vi "MAIN_save_merFISH_setpoint.vi"(3 "error in":errorcluster, 4 "Start acquisition":bool) -> (0 "error out":errorcluster, 1 "Next task":T2, 2 "QPD":T1)   [LabVIEW 2015]
uses:
  CONTROLS/Q_main_element.ctl
  GLOBAL/Global_FPGA.vi
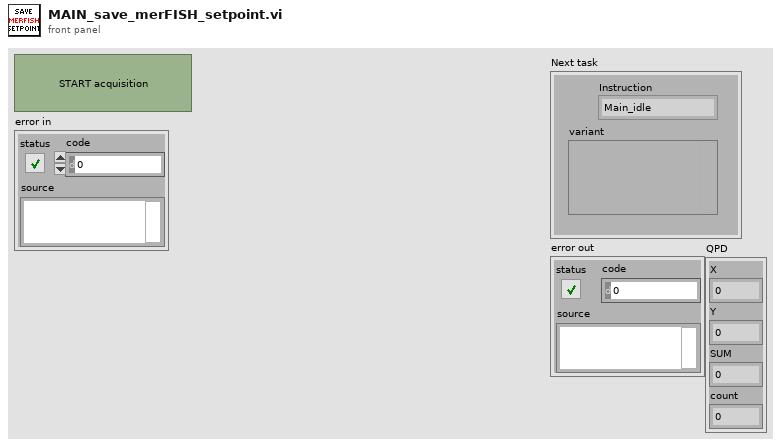
[diagram p1: front panel]
types:
  T1 = cluster{"X":sgl, "Y":sgl, "SUM":sgl, "count":u32}
  T2 = typedef "Q_main_element.ctl" = cluster{"variant":variant, "Instruction":enum16{"Main_idle", "Main_initialize", "Main_initialize_TDMS", "Main_initialize_Queue", "Main_error", "Main_DAQ_initialization_results", "Main_ASI_initialization_results", "Main_Piezo_initialization_results", "Main_Valve_initialization_results", "Main_Pump_initialization_results", "Main_CAMERA_initialization_results", "Main_FPGA_initialization_results", "Main_DAQ_error", "Main_ASI_error", "Main_Piezo_error", "Main_CAMERA_error", "Main_Valve_error", "Main_Pump_error", "Main_FPGA_error", "Main_start_acquiring", "Main_not_acquiring", "Main_acquiring", "Main_stop_acquiring", "Main_change_exposure", "Main_change_z_scan_parameters", "Main_define_ROI", "Main_define_mosaic", "Main_read_kinetic_time", "Main_cooler", "Main_read_temperature", "Main_save_XY", "Main_load_XY", "Main_discard_XY", "Main_move_to_XY", "Main_measure_QPD", "Main_autofocus_calibration", "Main_autofocus_initialization", "Main_autofocus_stop", "Main_save_PID", "Main_change_H_valve_position", "Main_two_way_valve", "Main_save_movie", "Main_init_single_scan", "Main_single_scan", "Main_stop_single_scan", "Main_merFISH_illumination_parameters", "Main_merFISH_buffer_probe_list", "Main_merFISH_injections_procedure", "Main_merFISH_save_setpoint", "Main_merFISH_DAPI_parameters", "Main_merFISH_Brightfield_parameters", "Main_merFISH_save_embryo_ROI", "Main_merFISH_init", "Main_merFISH_resume", "Main_merFISH_start_autofocus", "Main_merFISH_open_close_valve_merFISH", "Main_merFISH_open_close_valve_photobleaching", "Main_merFISH_hybridization", "Main_merFISH_move_to_ROI", "Main_merFISH_wait_stabilization", "Main_merFISH_move_to_REF", "Main_merFISH_scan", "Main_merFISH_photobleaching_injection", "Main_merFISH_photobleaching", "Main_merFISH_send_email", "Main_merFISH_close", "Main_STOP"}}
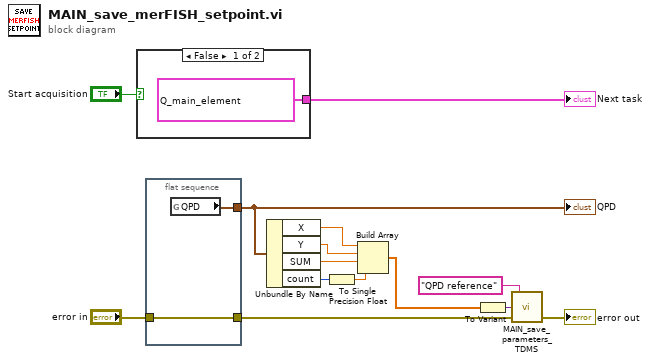
[diagram p0: block diagram]
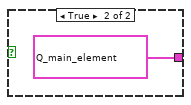
[diagram p2: hidden frame]
diagram:
  n1 = case shown="False" "Start acquisition" {
    tunnel: [T2 {"variant"=variant, "Instruction"=enum."Main_not_acquiring"} ("Q_main_element") T2 {"variant"=variant, "Instruction"=enum."Main_acquiring"} ("Q_main_element")] -> w10
    frame False {
    }
    frame True {
    }
  }
  "Next task" <- w10
  n2 = flat-sequence {
    tunnel: "error in" -> [w18]
    tunnel: [w18] -> w14
    tunnel: [w17] -> w7
    frame #0 {
      n3 = global read "Global_FPGA.vi" "QPD"() -> (w17:T1)
    }
  }
  n4 = Unbundle By Name(w7) -> ("X"=w6:sgl, "Y"=w5:sgl, "SUM"=w4:sgl, "count"=w2:u32)
  n5 = To Single Precision Float(number=w2) -> (single precision float=w3:sgl)
  n6 = Build Array(w6, w5, w4, w3) -> (w1:sgl[])
  n7 = To Variant(anything=w1) -> (Variant=w13:variant)
  n8 = call "MAIN_save_parameters_TDMS.vi"("error in"=w14, "Data"=w13, "Channel name"="QPD reference" ("group name")) -> ("error out"=→"error out":errorcluster)  [unwired: 2 in]
  "QPD" <- w7
